vi "Documentation.vi"   [LabVIEW 2019, in "Inst.Xeryon-Rotator.lvclass"]
uses:
  Inst.Xeryon-Rotator.lvclass
  <vilib>/JKI/JKI SMO/SMO/SMO.lvclass
  Typedefs/Inst.Xeryon-Rotator.getAll--Cluster.ctl
  Typedefs/Inst.Xeryon-Rotator.Configuration--Cluster.ctl
  Inst UI.Xeryon-Rotator/Inst UI.Xeryon-Rotator.lvclass
  Inst UI.Xeryon-Rotator/Inst UI.Xeryon-Rotator.UI--Cluster.ctl
  <userlib>/LevyLab/Instrument Framework/Instrument UI/Instrument UI.lvclass
  C:/Program Files (x86)/National Instruments/LabVIEW 2019/user.lib/LevyLab/Instrument Framework/Instrument Types/Cryostat/Instrument.Cryostat.lvclass
  C:/Program Files (x86)/National Instruments/LabVIEW 2019/user.lib/LevyLab/Instrument Framework/Instrument/Instrument.lvclass
  C:/Program Files (x86)/National Instruments/LabVIEW 2019/vi.lib/JKI/JKI SMO/SMO/SMO.lvclass
  Typedefs/Inst.Xeryon-Rotator.Commands--Enum.ctl
  <userlib>/LevyLab/Instrument Framework/Instrument/Instrument.lvclass
  <userlib>/LevyLab/Instrument Framework/Instrument/API/Instrument.sendMessageToProcess (string).vi
  C:/Program Files (x86)/National Instruments/LabVIEW 2019/user.lib/LevyLab/Instrument Framework/Instrument UI/Instrument UI.lvclass
  C:/Program Files (x86)/National Instruments/LabVIEW 2019/vi.lib/JKI/JKI SMO/SMO.UI/SMO.UI.lvclass
  <vilib>/JKI/JKI SMO/SMO.UI/SMO.UI.lvclass
  <userlib>/LevyLab/RemoteControl/RemoteControl/RemoteControl.lvclass
  fed5944e-40af-404e-90dd-c9efca414dd4.vi
types:
  T1 = typedef "Inst.Xeryon-Rotator.lvclass/Inst.Xeryon-Rotator.getAll--Cluster.ctl" = cluster{"Encoder position [selected units]":dbl, "Desired Position [selected units]":dbl, "Status":string, "SRNO":dbl, "SOFT":dbl, "STAT":dbl, "FREQ":dbl, "OFRQ":dbl, "CURR":dbl, "SYNC":dbl, "Encoder Position [enc. units]":dbl, "Desired Position [enc. units]":dbl, "TIME":dbl, "Index Found":bool, "Left Limit":bool, "Right Limit":bool, "Position Reached":bool}
  T2 = typedef "Inst.Xeryon-Rotator.lvclass/Inst.Xeryon-Rotator.Configuration--Cluster.ctl" = cluster{"Example Setting 1":dbl, "Example Setting 2":dbl, "Example Setting 3":string}
  T3 = typedef "Inst.Xeryon-Rotator.lvclass/Inst.Xeryon-Rotator.Commands--Enum.ctl" = enum16{"setAngle", "getAngle", "setState"}
  T4 = typedef "Inst UI.Xeryon-Rotator.lvclass/Inst UI.Xeryon-Rotator.UI--Cluster.ctl" = cluster{"Desired Position":dbl, "Desired Rate":dbl}
  T5 = typedef "Instrument.lvlib/Instrument.lvclass/PublicEvents--Cluster.ctl" = cluster{"MessageFromProcess":refnum<user-event>}
  T6 = typedef "Instrument.lvlib/Instrument.lvclass/PrivateEvents--Cluster.ctl" = cluster{"MessageToProcess":refnum<user-event>, "LogData":refnum<user-event>, "LogDataMultiline":refnum<user-event>}
  T7 = typedef "Inst.Xeryon-Rotator.lvclass/PublicEvents--Cluster.ctl" = cluster{"MessageFromProcess":refnum<user-event>}
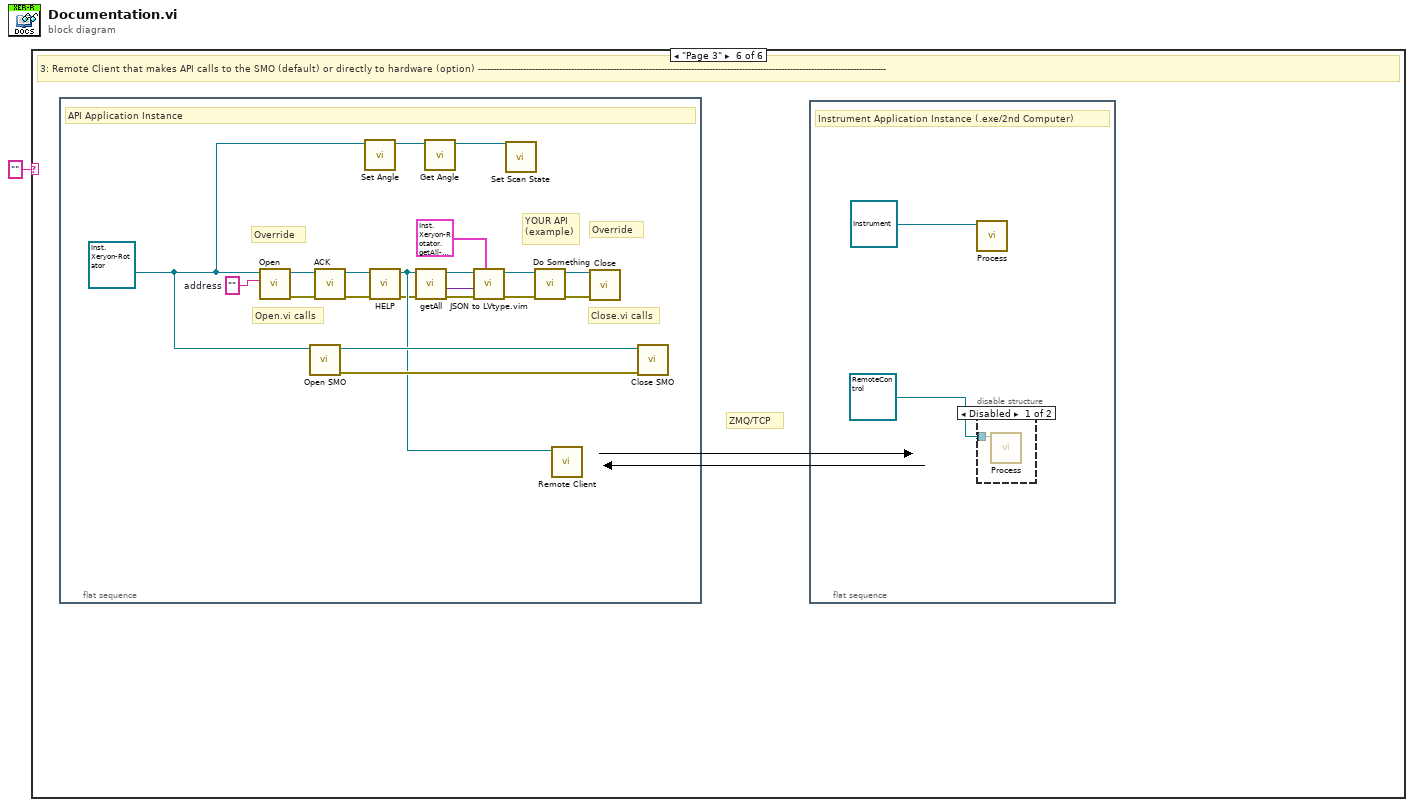
[diagram p0: block diagram]
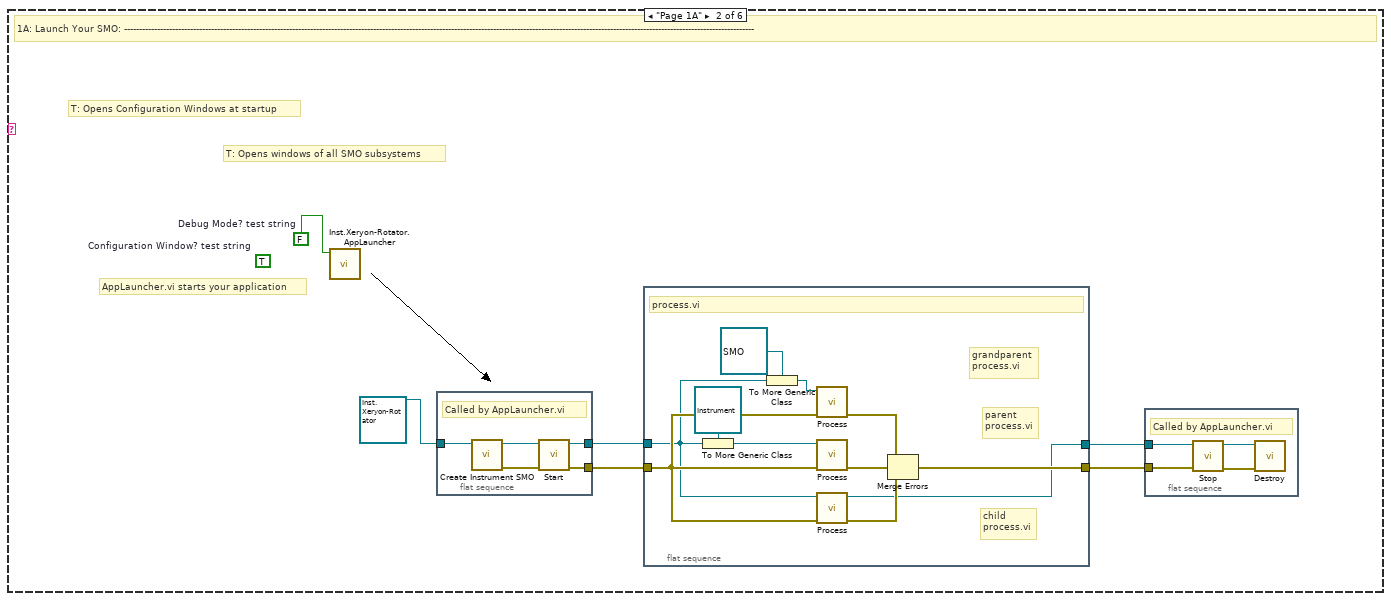
[diagram p3: hidden frame]
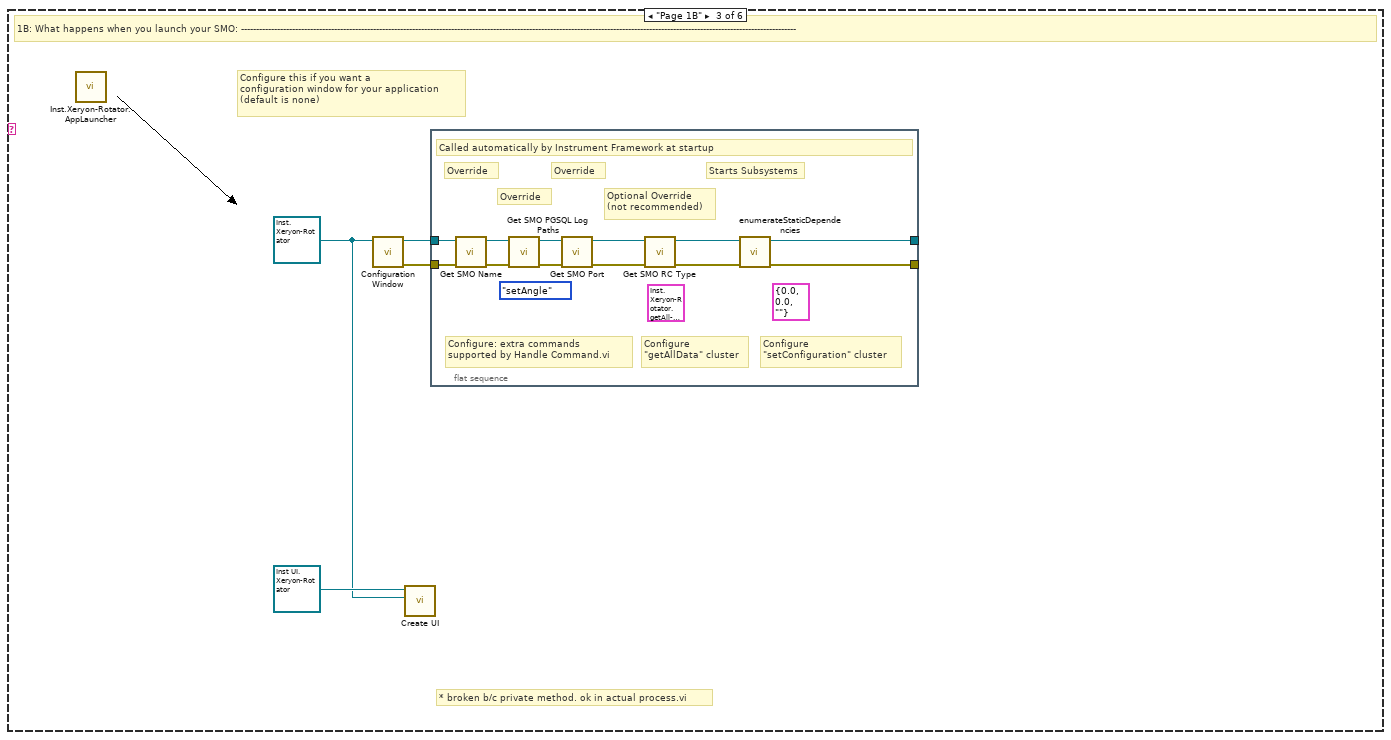
[diagram p4: hidden frame]
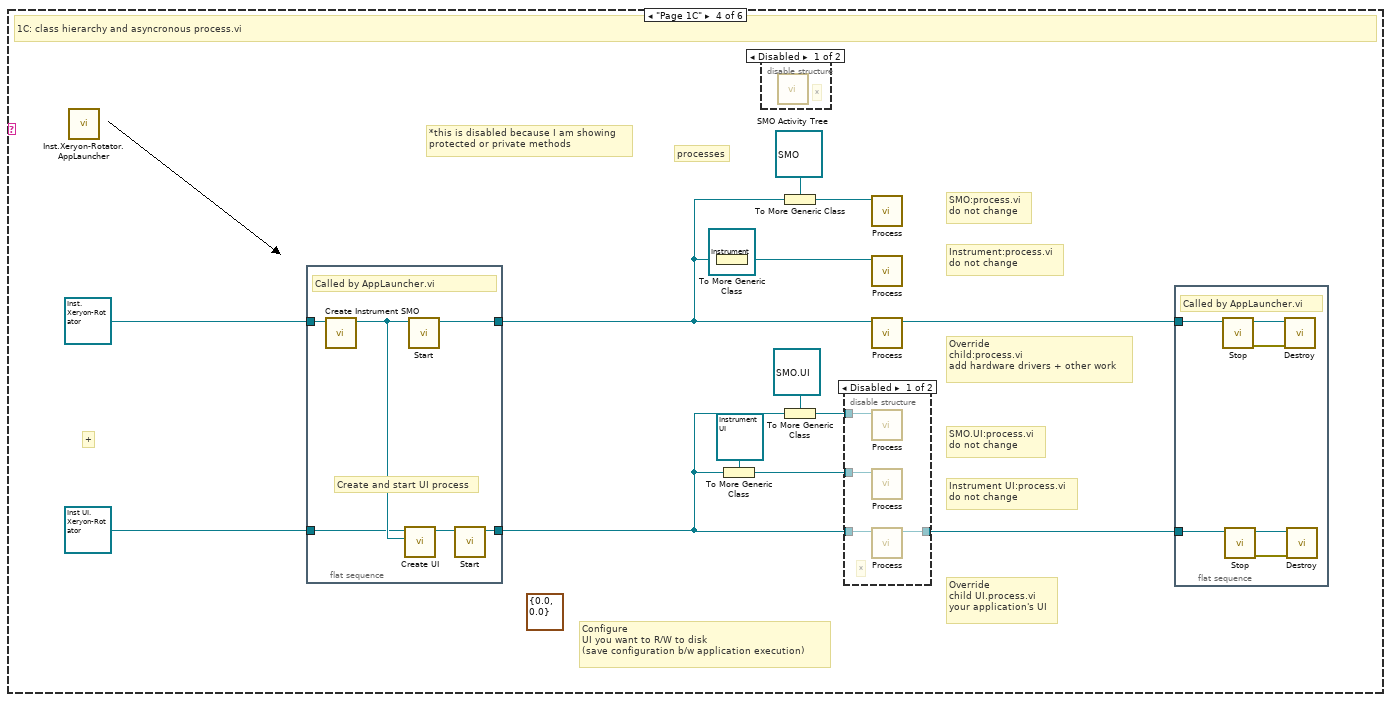
[diagram p5: hidden frame]
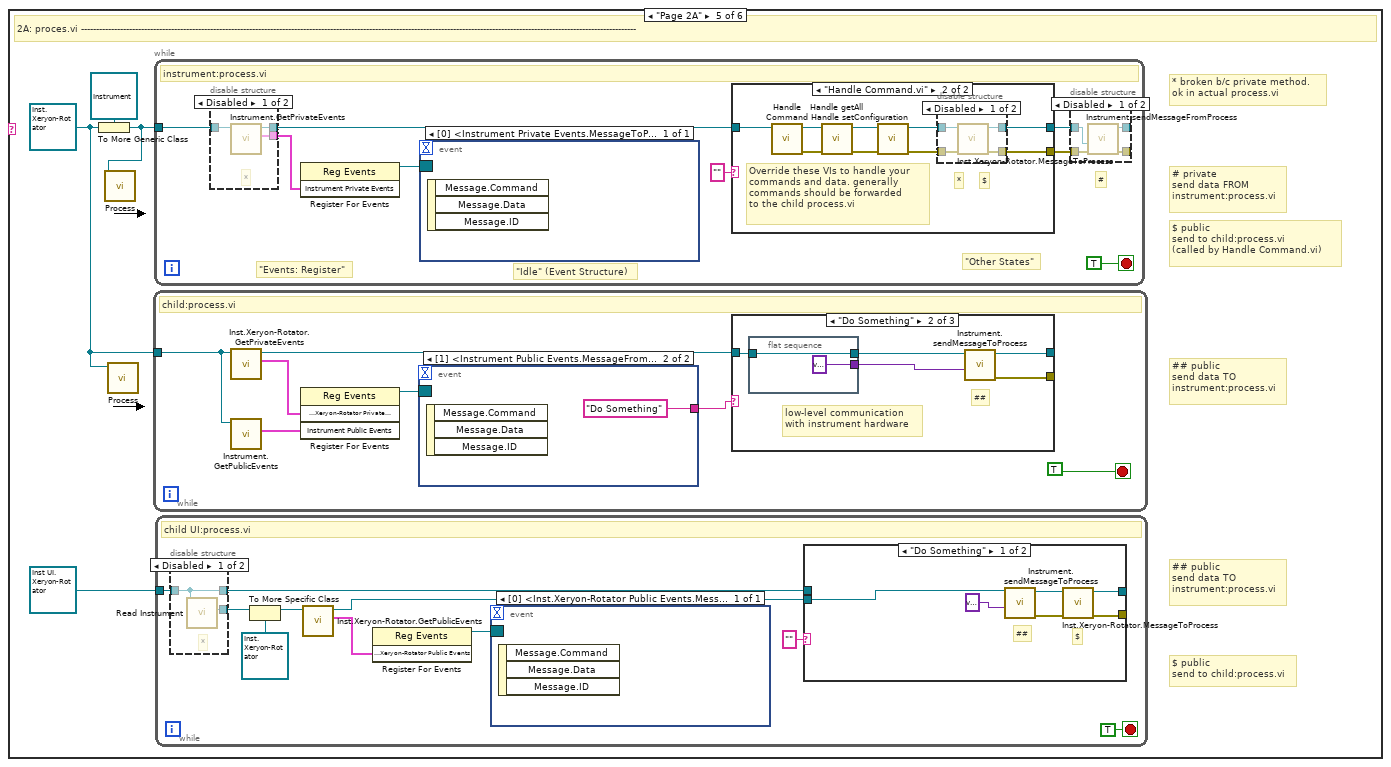
[diagram p8: hidden frame]
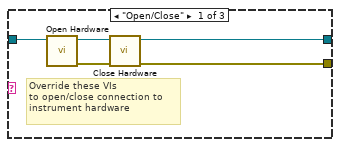
[diagram p11: hidden frame]
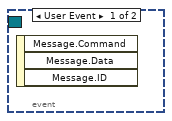
[diagram p13: hidden frame]
diagram:
  n1 = case shown="\"Page 3\"" "" {
    frame Default {
    }
    frame "Page 1A" {
      (unwired) TRUE  # Configuration Window? test string
      w7 = FALSE  # Debug Mode? test string
      # "AppLauncher.vi starts your application"
      # "T: Opens windows of all SMO subsystems"
      # "T: Opens Configuration Windows at startup"
      # "1A: Launch Your SMO: ------------------------------------------------------------------------------------------------------------------------------------------------------------------------------------------------------------------"
      n2 = call "Inst.Xeryon-Rotator.AppLauncher.vi"("Debug Mode"=w7) -> ()  [unwired: 10 in, 1 out]
      n3 = flat-sequence {
        tunnel: [w25] -> w3
        tunnel: [w24] -> w5
        tunnel: refnum<class "Inst.Xeryon-Rotator.lvclass"> refnum ("Instrument.Template.lvclass") -> [w23]
        frame #0 {
          # "Called by AppLauncher.vi"
          n4 = call <userlib>:"Create Instrument SMO.vi"("Instrument in"=w23) -> ("error out"=w26:errorcluster, "Instrument out"=w27:refnum<class "Inst.Xeryon-Rotator.lvclass">)  [unwired: 9 in]
          n5 = call <vilib>:"Start.vi"("error in (no error)"=w26, "SMO"=w27) -> ("error out"=w24:errorcluster, "SMO out"=w25:refnum<class "Inst.Xeryon-Rotator.lvclass">)  [unwired: 8 in]
        }
      }
      n6 = flat-sequence {
        tunnel: [w18] -> w6
        tunnel: w5 -> [w16]
        tunnel: [w10] -> w4
        tunnel: w3 -> [w9]
        frame #0 {
          # "child\nprocess.vi"
          # "grandparent\nprocess.vi"
          # "parent\nprocess.vi"
          # "process.vi"
          n7 = To More Generic Class(target class=refnum<class "Instrument.lvclass"> refnum ("Instrument"), reference=w9) -> (generic class reference=w15:refnum<class "Instrument.lvclass">)
          n8 = To More Generic Class(target class=refnum<class "SMO.lvclass"> refnum ("SMO"), reference=w9) -> (generic class reference=w17:refnum<class "SMO.lvclass">)
          n9 = call-dynamic "Process.vi"("error in"=w16, "SMO"=w17) -> ("error out"=w11:errorcluster)  [unwired: 8 in, 1 out]
          n10 = call-dynamic "Process.vi"("error in"=w16, "Instrument"=w15) -> ("error out"=w13:errorcluster)  [unwired: 8 in, 1 out]
          n11 = call-dynamic "Process.vi"("error in"=w16, "Inst.Xeryon-Rotator"=w9) -> ("error out"=w12:errorcluster, "Inst.Xeryon-Rotator out"=w10:refnum<class "Inst.Xeryon-Rotator.lvclass">)  [unwired: 8 in]
          n12 = Merge Errors(w11, w13, w12) -> (w18:errorcluster)
        }
      }
      n13 = flat-sequence {
        tunnel: w4 -> [w20]
        tunnel: w6 -> [w19]
        frame #0 {
          # "Called by AppLauncher.vi"
          n14 = call <vilib>:"Stop.vi"("error in (no error)"=w19, "SMO"=w20) -> ("error out"=w22:errorcluster, "SMO out"=w21:refnum<class "Inst.Xeryon-Rotator.lvclass">)  [unwired: 8 in]
          n15 = call <vilib>:"Destroy.vi"("error in (no error)"=w22, "SMO"=w21) -> ()  [unwired: 9 in, 1 out]
        }
      }
    }
    frame "Page 1B" {
      w28 = refnum<class "Inst.Xeryon-Rotator.lvclass"> refnum ("Instrument.Template.lvclass")
      # "* broken b/c private method. ok in actual process.vi"
      # "Configure this if you want a\nconfiguration window for your application\n(default is none)"
      # "1B: What happens when you launch your SMO: -----------------------------------------------------------------------------------------------------------------------------------------------------------------------------------------"
      n16 = call "Inst.Xeryon-Rotator.AppLauncher.vi"() -> ()  [unwired: 11 in, 1 out]
      n17 = call-dynamic "Configuration Window.vi"("Inst.Xeryon-Rotator in"=w28) -> ("error out"=w30:errorcluster, "Inst.Xeryon-Rotator out"=w31:refnum<class "Inst.Xeryon-Rotator.lvclass">)  [unwired: 9 in]
      n18 = call <userlib>:"Create UI.vi"("Instrument in"=w28, "Instrument UI"=refnum<class "Inst UI.Xeryon-Rotator.lvclass"> refnum ("Instrument UI.Template.lvclass")) -> ()  [unwired: 8 in, 2 out]
      n19 = flat-sequence {
        tunnel: w31 -> [w39]
        tunnel: w30 -> [w34]
        tunnel: [w33] -> _
        tunnel: [w32] -> _
        frame #0 {
          (unwired) T2 {"Example Setting 1"=0.0, "Example Setting 2"=0.0, "Example Setting 3"=""} ("Configuration")
          (unwired) T1 {"Encoder position [selected units]"=0.0, "Desired Position [selected units]"=0.0, "Status"="", "SRNO"=0.0, "SOFT"=0.0, "STAT"=0.0, "FREQ"=0.0, "OFRQ"=0.0, "CURR"=0.0, "SYNC"=0.0, "Encoder Position [enc. units]"=0.0, "Desired Position [enc. units]"=0.0, "TIME"=0.0, "Index Found"=FALSE, "Left Limit"=FALSE, "Right Limit"=FALSE, "Position Reached"=FALSE} ("getAll")
          (unwired) Inst.Xeryon-Rotator.Commands--Enum."setAngle" ("Commands")
          # "Configure\n\"setConfiguration\" cluster"
          # "Configure\n\"getAllData\" cluster"
          # "Configure: extra commands\nsupported by Handle Command.vi"
          # "Starts Subsystems"
          # "Override"
          # "Override"
          # "Override"
          # "Optional Override\n(not recommended)"
          # "Called automatically by Instrument Framework at startup"
          n20 = call-dynamic "Get SMO Name.vi"("error in (no error)"=w34, "Inst.Xeryon-Rotator in"=w39) -> ("error out"=w37:errorcluster, "Inst.Xeryon-Rotator out"=w38:refnum<class "Inst.Xeryon-Rotator.lvclass">)  [unwired: 7 in, 1 out]
          n21 = call-dynamic "Get SMO PGSQL Log Paths.vi"("error in (no error)"=w37, "Inst.Xeryon-Rotator in"=w38) -> ("error out"=w35:errorcluster, "Inst.Xeryon-Rotator out"=w36:refnum<class "Inst.Xeryon-Rotator.lvclass">)  [unwired: 7 in, 1 out]
          n22 = call-dynamic "Get SMO Port.vi"("error in (no error)"=w35, "Inst.Xeryon-RotatorInstrument in"=w36) -> ("error out"=w40:errorcluster, "Inst.Xeryon-RotatorInstrument out"=w41:refnum<class "Inst.Xeryon-Rotator.lvclass">)  [unwired: 7 in, 1 out]
          n23 = call-dynamic "Get SMO RC Type.vi"("error in (no error)"=w40, "Instrument in"=w41) -> ("error out"=w42:errorcluster, "Instrument out"=w43:refnum<class "Inst.Xeryon-Rotator.lvclass">)  [unwired: 7 in, 1 out]
          n24 = call-dynamic "enumerateStaticDependencies.vi"("error in (no error)"=w42, "Instrument"=w43) -> ("error out"=w33:errorcluster, "Instrument out"=w32:refnum<class "Inst.Xeryon-Rotator.lvclass">)  [unwired: 7 in, 1 out]
        }
      }
    }
    frame "Page 1C" {
      (unwired) T4 {"Desired Position"=0.0, "Desired Rate"=0.0} ("UI")
      # "processes"
      # "SMO.UI:process.vi\ndo not change"
      # "Instrument UI:process.vi\ndo not change"
      # "Override\nchild:process.vi\nadd hardware drivers + other work"
      # "SMO:process.vi\ndo not change"
      # "Instrument:process.vi\ndo not change"
      # "*this is disabled because I am showing\nprotected or private methods"
      # "Configure\nUI you want to R/W to disk\n(save configuration b/w application execution)"
      # "Override\nchild UI.process.vi\nyour application's UI"
      # "+"
      # "1C: class hierarchy and asyncronous process.vi"
      n25 = call "Inst.Xeryon-Rotator.AppLauncher.vi"() -> ()  [unwired: 11 in, 1 out]
      n26 = flat-sequence {
        tunnel: [w73] -> w56
        tunnel: refnum<class "Inst.Xeryon-Rotator.lvclass"> refnum ("Instrument.Template.lvclass") -> [w72]
        tunnel: refnum<class "Inst UI.Xeryon-Rotator.lvclass"> refnum ("Instrument UI.Template.lvclass") -> [w70]
        tunnel: [w68] -> w54
        frame #0 {
          # "Create and start UI process"
          # "Called by AppLauncher.vi"
          n27 = call <userlib>:"Create Instrument SMO.vi"("Instrument in"=w72) -> ("Instrument out"=w71:refnum<class "Inst.Xeryon-Rotator.lvclass">)  [unwired: 9 in, 1 out]
          n28 = call <userlib>:"Create UI.vi"("Instrument in"=w71, "Instrument UI"=w70) -> ("Instrument UI out"=w69:refnum<class "Inst UI.Xeryon-Rotator.lvclass">)  [unwired: 8 in, 1 out]
          n29 = call <vilib>:"Start.vi"("SMO"=w71) -> ("SMO out"=w73:refnum<class "Inst.Xeryon-Rotator.lvclass">)  [unwired: 9 in, 1 out]
          n30 = call <vilib>:"Start.vi"("SMO"=w69) -> ("SMO out"=w68:refnum<class "Inst UI.Xeryon-Rotator.lvclass">)  [unwired: 9 in, 1 out]
        }
      }
      n31 = To More Generic Class(target class=refnum<class "Instrument.lvclass"> refnum ("Instrument"), reference=w56) -> (generic class reference=w51:refnum<class "Instrument.lvclass">)
      n32 = To More Generic Class(target class=refnum<class "Instrument UI.lvclass"> refnum ("Instrument UI"), reference=w54) -> (generic class reference=w47:refnum<class "Instrument UI.lvclass">)
      n33 = disable-structure shown="Disabled" {
        frame Disabled {
          # "*"
          n34 = call <vilib>:"SMO Activity Tree.vi"() -> ()  [unwired: 12 in]
        }
        frame Enabled {
        }
      }
      n35 = To More Generic Class(target class=refnum<class "SMO.lvclass"> refnum ("SMO"), reference=w56) -> (generic class reference=w52:refnum<class "SMO.lvclass">)
      n36 = To More Generic Class(target class=refnum<class "SMO.UI.lvclass"> refnum ("SMO.UI"), reference=w54) -> (generic class reference=w45:refnum<class "SMO.UI.lvclass">)
      n37 = disable-structure shown="Disabled" {
        disable-tunnel: w54 -> [w61 _]
        disable-tunnel: [w60 _] -> w53
        disable-tunnel: w47 -> [w59 _]
        disable-tunnel: w45 -> [w58 _]
        frame Disabled {
          # "*"
          n38 = call-dynamic "Process.vi"("SMO.UI"=w58) -> ()  [unwired: 9 in, 2 out]
          n39 = call-dynamic "Process.vi"("Instrument UI in"=w59) -> ()  [unwired: 9 in, 2 out]
          n40 = call-dynamic "Process.vi"("Inst UI.Xeryon-Rotator"=w61) -> ("Inst UI.Xeryon-Rotator out"=w60:refnum<class "Inst UI.Xeryon-Rotator.lvclass">)  [unwired: 9 in, 1 out]
        }
        frame Enabled {
        }
      }
      n41 = call-dynamic "Process.vi"("SMO"=w52) -> ()  [unwired: 9 in, 2 out]
      n42 = call-dynamic "Process.vi"("Instrument"=w51) -> ()  [unwired: 9 in, 2 out]
      n43 = call-dynamic "Process.vi"("Inst.Xeryon-Rotator"=w56) -> ("Inst.Xeryon-Rotator out"=w57:refnum<class "Inst.Xeryon-Rotator.lvclass">)  [unwired: 9 in, 1 out]
      n44 = flat-sequence {
        tunnel: w57 -> [w65]
        tunnel: w53 -> [w63]
        frame #0 {
          # "Called by AppLauncher.vi"
          n45 = call <vilib>:"Stop.vi"("SMO"=w65) -> ("error out"=w67:errorcluster, "SMO out"=w66:refnum<class "Inst.Xeryon-Rotator.lvclass">)  [unwired: 9 in]
          n46 = call <vilib>:"Stop.vi"("SMO"=w63) -> ("error out"=w64:errorcluster, "SMO out"=w62:refnum<class "Inst UI.Xeryon-Rotator.lvclass">)  [unwired: 9 in]
          n47 = call <vilib>:"Destroy.vi"("error in (no error)"=w67, "SMO"=w66) -> ()  [unwired: 9 in, 1 out]
          n48 = call <vilib>:"Destroy.vi"("error in (no error)"=w64, "SMO"=w62) -> ()  [unwired: 9 in, 1 out]
        }
      }
    }
    frame "Page 2A" {
      w74 = refnum<class "Inst.Xeryon-Rotator.lvclass"> refnum ("Instrument.Template.lvclass")
      # "## public\nsend data TO\ninstrument:process.vi"
      # "$ public\nsend to child:process.vi"
      # "## public\nsend data TO\ninstrument:process.vi"
      # "$ public\nsend to child:process.vi\n(called by Handle Command.vi)"
      # "# private\nsend data FROM\ninstrument:process.vi"
      # "* broken b/c private method.\nok in actual process.vi"
      # "2A: proces.vi -----------------------------------------------------------------------------------------------------------------------------------------------------------------------------------------"
      n49 = To More Generic Class(target class=refnum<class "Instrument.lvclass"> refnum ("Instrument"), reference=w74) -> (generic class reference=w75:refnum<class "Instrument.lvclass">)
      n50 = call-dynamic "Process.vi"("Instrument"=w75) -> ()  [unwired: 9 in, 2 out]
      n51 = call-dynamic "Process.vi"("Inst.Xeryon-Rotator"=w74) -> ()  [unwired: 9 in, 2 out]
      n52 = while {
        tunnel: w74 -> [w100]
        stop <- TRUE stop-if-true
        # "child:process.vi"
        n53 = call "Inst.Xeryon-Rotator.GetPrivateEvents.vi"("Inst.Xeryon-Rotator in"=w100) -> ("Inst.Xeryon-Rotator Private Events"=w104:cluster{"MessageToProcess":refnum<user-event>}, "Inst.Xeryon-Rotator out"=w102:refnum<class "Inst.Xeryon-Rotator.lvclass">)  [unwired: 8 in, 1 out]
        n54 = call <userlib>:"Instrument.GetPublicEvents.vi"("Instrument"=w100) -> ("Instrument Public Events"=w101:T5)  [unwired: 8 in, 2 out]
        n55 = register-events(w104, w101) -> (reference out=w103:refnum<event-registration>)  [unwired: 2 in, 1 out]
        n56 = event shown="[1] <Instrument Public Events.MessageFromProcess>: User Event" {
          selector: w103 -> [_ _]
          dyn-events: _ -> [_ _]
          timeout: _ -> [_ _]
          tunnel: [_ "Do Something"] -> w98
          event User Event {
            n57 = event-data() -> ()  [unwired: 1 in, 3 out]
          }
          event User Event {
            n58 = event-data() -> ()  [unwired: 1 in, 3 out]
          }
        }
        n59 = case shown="\"Do Something\"" w98 {
          tunnel: w102 -> [w107 w112 w117]
          tunnel: [w106 w114 w117] -> _
          tunnel: [w105 w113 _] -> _
          frame "Open/Close" {
            # "Override these VIs\nto open/close connection to\ninstrument hardware"
            n60 = call-dynamic "Open Hardware.vi"("Inst.Xeryon-Rotator in"=w107) -> ("error out"=w109:errorcluster, "Inst.Xeryon-Rotator out"=w108:refnum<class "Inst.Xeryon-Rotator.lvclass">)  [unwired: 9 in]
            n61 = call-dynamic "Close Hardware.vi"("error in (no error)"=w109, "Inst.Xeryon-Rotator in"=w108) -> ("error out"=w105:errorcluster, "Inst.Xeryon-Rotator out"=w106:refnum<class "Inst.Xeryon-Rotator.lvclass">)  [unwired: 8 in]
          }
          frame "Do Something" {
            # "##"
            # "low-level communication\nwith instrument hardware"
            n62 = flat-sequence {
              tunnel: w112 -> [w116]
              tunnel: [w116] -> w111
              tunnel: [variant ("Data")] -> w110
              frame #0 {
              }
            }
            n63 = call-poly <userlib>:"Instrument.sendMessageToProcess.vi"("Data"=w110, "Instrument"=w111) -> ("error out"=w113:errorcluster, "Instrument out"=w114:refnum<class "Inst.Xeryon-Rotator.lvclass">)  [unwired: 8 in]
          }
          frame Default {
          }
        }
      }
      n64 = while {
        tunnel: w75 -> [w125]
        stop <- TRUE stop-if-true
        # "#"
        # "\"Other States\""
        # "\"Idle\" (Event Structure)"
        # "\"Events: Register\""
        # "instrument:process.vi"
        n65 = disable-structure shown="Disabled" {
          disable-tunnel: w125 -> [w149 w150]
          disable-tunnel: [w148 w150] -> w124
          disable-tunnel: [w147 _] -> w123
          frame Disabled {
            # "*"
            n66 = call <userlib>:"Instrument.GetPrivateEvents.vi"("Instrument"=w149) -> ("Instrument Private Events"=w147:T6, "Instrument out"=w148:refnum<class "Instrument.lvclass">)  [unwired: 8 in, 1 out]
          }
          frame Enabled {
          }
        }
        n67 = register-events(w123) -> (reference out=w122:refnum<event-registration>)  [unwired: 2 in, 1 out]
        n68 = event shown="[0] <Instrument Private Events.MessageToProcess>: User Event" {
          selector: w122 -> [_]
          dyn-events: _ -> [_]
          timeout: _ -> [_]
          event User Event {
            n69 = event-data() -> ()  [unwired: 1 in, 3 out]
          }
        }
        n70 = case shown="\"Handle Command.vi\"" "" {
          tunnel: w124 -> [w131 w140]
          tunnel: [w131 w134] -> w121
          tunnel: [_ w133] -> w120
          frame Default {
          }
          frame "Handle Command.vi" {
            # "*"
            # "$"
            # "Override these VIs to handle your\ncommands and data. generally \ncommands should be forwarded\nto the child process.vi"
            n71 = call-dynamic "Handle Command.vi"("Instrument in"=w140) -> ("error out"=w136:errorcluster, "Instrument out"=w139:refnum<class "Instrument.lvclass">)  [unwired: 7 in, 2 out]
            n72 = call-dynamic "Handle getAll.vi"("error in (no error)"=w136, "Instrument in"=w139) -> ("error out"=w137:errorcluster, "Instrument out"=w138:refnum<class "Instrument.lvclass">)  [unwired: 7 in, 1 out]
            n73 = call-dynamic "Handle setConfiguration.vi"("error in (no error)"=w137, "Instrument in"=w138) -> ("error out"=w132:errorcluster, "Instrument out"=w135:refnum<class "Instrument.lvclass">)  [unwired: 8 in]
            n74 = disable-structure shown="Disabled" {
              disable-tunnel: w135 -> [w144 w146]
              disable-tunnel: [w143 w146] -> w134
              disable-tunnel: [w142 w145] -> w133
              disable-tunnel: w132 -> [w141 w145]
              frame Disabled {
                n75 = call "Inst.Xeryon-Rotator.MessageToProcess.vi"("error in (no error)"=w141, "Inst.Xeryon-Rotator in"=w144) -> ("error out"=w142:errorcluster, "Inst.Xeryon-Rotator out"=w143:refnum<class "Inst.Xeryon-Rotator.lvclass">)  [unwired: 8 in]
              }
              frame Enabled {
              }
            }
          }
        }
        n76 = disable-structure shown="Disabled" {
          disable-tunnel: w121 -> [w130 _]
          disable-tunnel: w120 -> [w129 _]
          disable-tunnel: [w128 _] -> _
          disable-tunnel: [w127 _] -> _
          frame Disabled {
            n77 = call <userlib>:"Instrument.sendMessageFromProcess.vi"("error in (no error)"=w129, "Data"=w130) -> ("error out"=w128:errorcluster, "Instrument out"=w127:refnum<class "Instrument.lvclass">)  [unwired: 8 in]
          }
          frame Enabled {
          }
        }
      }
      n78 = while {
        tunnel: refnum<class "Inst UI.Xeryon-Rotator.lvclass"> refnum ("Instrument UI.Template.lvclass") -> [w86]
        stop <- TRUE stop-if-true
        # "child UI:process.vi"
        n79 = disable-structure shown="Disabled" {
          disable-tunnel: w86 -> [w95 w97]
          disable-tunnel: [w96 _] -> w84
          disable-tunnel: [w95 w97] -> w80
          frame Disabled {
            # "*"
            n80 = call <userlib>:"Read Instrument.vi"("Instrument UI in"=w95) -> ("Instrument"=w96:refnum<class "Instrument.lvclass">)  [unwired: 8 in, 2 out]
          }
          frame Enabled {
          }
        }
        n81 = To More Specific Class(target class=refnum<class "Inst.Xeryon-Rotator.lvclass"> refnum ("Instrument.Template.lvclass"), reference=w84) -> (specific class reference=w83:refnum<class "Inst.Xeryon-Rotator.lvclass">)  [unwired: 1 in, 1 out]
        n82 = call "Inst.Xeryon-Rotator.GetPublicEvents.vi"("Inst.Xeryon-Rotator in"=w83) -> ("Inst.Xeryon-Rotator Public Events"=w81:T7, "Inst.Xeryon-Rotator out"=w79:refnum<class "Inst.Xeryon-Rotator.lvclass">)  [unwired: 8 in, 1 out]
        n83 = register-events(w81) -> (reference out=w82:refnum<event-registration>)  [unwired: 2 in, 1 out]
        n84 = event shown="[0] <Inst.Xeryon-Rotator Public Events.MessageFromProcess>: User Event" {
          selector: w82 -> [_]
          dyn-events: _ -> [_]
          timeout: _ -> [_]
          event User Event {
            n85 = event-data() -> ()  [unwired: 1 in, 3 out]
          }
        }
        n86 = case shown="\"Do Something\"" "" {
          tunnel: w80 -> [_ _]
          tunnel: [w90 w94] -> _
          tunnel: [w89 _] -> _
          tunnel: w79 -> [w91 w94]
          frame "Do Something" {
            # "##"
            # "$"
            n87 = call-poly <userlib>:"Instrument.sendMessageToProcess.vi"("Data"=variant, "Instrument"=w91) -> ("error out"=w88:errorcluster, "Instrument out"=w92:refnum<class "Inst.Xeryon-Rotator.lvclass">)  [unwired: 8 in]
            n88 = call "Inst.Xeryon-Rotator.MessageToProcess.vi"("error in (no error)"=w88, "Inst.Xeryon-Rotator in"=w92) -> ("error out"=w89:errorcluster, "Inst.Xeryon-Rotator out"=w90:refnum<class "Inst.Xeryon-Rotator.lvclass">)  [unwired: 8 in]
          }
          frame Default {
          }
        }
      }
    }
    frame "Page 3" {
      # "ZMQ/TCP"
      # "3: Remote Client that makes API calls to the SMO (default) or directly to hardware (option) ----------------------------------------------------------------------------------------------------------------------------------------"
      n89 = flat-sequence {
        frame #0 {
          w165 = ""  # address
          w161 = refnum<class "Inst.Xeryon-Rotator.lvclass"> refnum ("Instrument.Template.lvclass")
          # "Close.vi calls"
          # "Open.vi calls"
          # "YOUR API\n(example)"
          # "Override"
          # "Override"
          # "API Application Instance"
          n90 = call-dynamic "Open.vi"("address"=w165, "Inst.Xeryon-Rotator in"=w161) -> ("error out"=w172:errorcluster, "Inst.Xeryon-Rotator out"=w171:refnum<class "Inst.Xeryon-Rotator.lvclass">)  [unwired: 8 in]
          n91 = call <userlib>:"Open SMO.vi"("Instrument in"=w161) -> ("error out"=w163:errorcluster, "Instrument out"=w164:refnum<class "Inst.Xeryon-Rotator.lvclass">)  [unwired: 9 in]
          n92 = call <userlib>:"ACK.vi"("error in (no error)"=w172, "Instrument in"=w171) -> ("error out"=w170:errorcluster, "Instrument out"=w169:refnum<class "Inst.Xeryon-Rotator.lvclass">)  [unwired: 7 in, 1 out]
          n93 = call-dynamic "Set Angle.vi"("Inst.Xeryon-Rotator in"=w161) -> ("Inst.Xeryon-Rotator out"=w162:refnum<class "Inst.Xeryon-Rotator.lvclass">)  [unwired: 9 in, 1 out]
          n94 = call <userlib>:"HELP.vi"("error in (no error)"=w170, "Instrument in"=w169) -> ("error out"=w158:errorcluster, "Instrument in"=w159:refnum<class "Inst.Xeryon-Rotator.lvclass">)  [unwired: 7 in, 1 out]
          n95 = call <userlib>:"getAll.vi"("error in (no error)"=w158, "Instrument in"=w159) -> ("error out"=w155:errorcluster, "getAll"=w156:variant, "Instrument out"=w166:refnum<class "Inst.Xeryon-Rotator.lvclass">)  [unwired: 7 in]
          n96 = call-dynamic "Get Angle.vi"("Inst.Xeryon-Rotator in"=w162) -> ("Inst.Xeryon-Rotator out"=w160:refnum<class "Inst.Xeryon-Rotator.lvclass">)  [unwired: 7 in, 3 out]
          n97 = call "JSON to LVtype.vim"("type"=T1 {"Encoder position [selected units]"=0.0, "Desired Position [selected units]"=0.0, "Status"="", "SRNO"=0.0, "SOFT"=0.0, "STAT"=0.0, "FREQ"=0.0, "OFRQ"=0.0, "CURR"=0.0, "SYNC"=0.0, "Encoder Position [enc. units]"=0.0, "Desired Position [enc. units]"=0.0, "TIME"=0.0, "Index Found"=FALSE, "Left Limit"=FALSE, "Right Limit"=FALSE, "Position Reached"=FALSE} ("getAll"), "error in (no error)"=w155, "JSON Data in"=w156) -> ("error out"=w154:errorcluster)  [unwired: 7 in, 1 out]
          n98 = call-dynamic "Set Scan State.vi"("Inst.Xeryon-Rotator in"=w160) -> ()  [unwired: 9 in, 2 out]
          n99 = call-dynamic "Do Something.vi"("error in (no error)"=w154, "Inst.Xeryon-Rotator in"=w166) -> ("error out"=w167:errorcluster, "Inst.Xeryon-Rotator out"=w168:refnum<class "Inst.Xeryon-Rotator.lvclass">)  [unwired: 8 in]
          n100 = call <userlib>:"Remote Client.vi"("Instrument in"=w159) -> ()  [unwired: 7 in, 4 out]
          n101 = call-dynamic "Close.vi"("error in (no error)"=w167, "Inst.Xeryon-Rotator in"=w168) -> ()  [unwired: 8 in, 2 out]
          n102 = call <userlib>:"Close SMO.vi"("error in (no error)"=w163, "Instrument in"=w164) -> ()  [unwired: 8 in, 2 out]
        }
      }
      n103 = flat-sequence {
        frame #0 {
          # "Instrument Application Instance (.exe/2nd Computer)"
          n104 = call-dynamic "Process.vi"("Instrument"=refnum<class "Instrument.lvclass"> refnum) -> ()  [unwired: 9 in, 2 out]
          n105 = disable-structure shown="Disabled" {
            disable-tunnel: refnum<class "RemoteControl.lvclass"> refnum ("RemoteControl out") -> [w153 _]
            frame Disabled {
              n106 = call-dynamic "Process.vi"("RemoteControl"=w153) -> ()  [unwired: 9 in, 2 out]
            }
            frame Enabled {
            }
          }
        }
      }
    }
  }
